vi "ClsCloseConnection.vi"(8 "error in (no error)":errorcluster, 11 "Connection In":u32) -> (0 "error out":errorcluster)   [LabVIEW 2015]
doc: "Close Connection:\n\nYou must use this vi to disconnect from the device after finishing your device usage. \n\nConnection In[Input]: the connection handle to be disconnected from which is initially created by Open Connection subVI."
uses:
  dependent dlls/CHRocodileDLL.dll
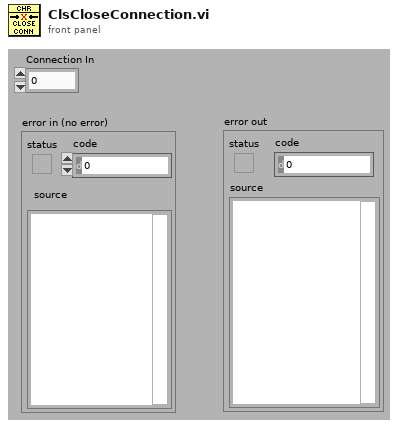
[diagram p1: front panel]
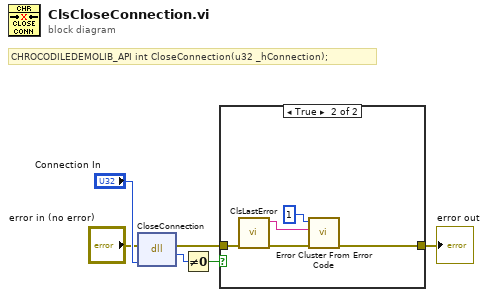
[diagram p0: block diagram]
diagram:
  # "CHROCODILEDEMOLIB_API int CloseConnection(u32 _hConnection);"
  n1 = dll-call lib="W:/Drop Impact Teststand/dependent dlls/CHRocodileDLL.*" fn="CloseConnection"(error in="error in (no error)", "_hConnection"="Connection In") -> (error out=w1:errorcluster, "return type"=w2:i32)  [unwired: 3 in, 1 out]
  n2 = Not Equal To 0?(x=w2) -> (x != 0?=w4:bool)
  n3 = case shown="True" w4 {
    tunnel: [w7 w10] -> w3
    tunnel: w1 -> [w7 w9]
    frame False {
    }
    frame True {
      n4 = call "ClsLastError.vi"("error in (no error)"=w9) -> ("error out"=w8:errorcluster, "Error Message"=w12:string)  [unwired: 9 in]
      n5 = call <vilib>:"Error Cluster From Error Code.vi"("error in (no error)"=w8, "error message (\"\")"=w12, "error code (0)"=1) -> ("error out"=w10:errorcluster)  [unwired: 6 in]
    }
  }
  "error out" <- w3
